vi "Check State.vi"(8 "error in (no error)":errorcluster, 11 "Shutter in":refnum<class "Shutter.lvclass">) -> (0 "error out":errorcluster, 3 "Shutter out":refnum<class "Shutter.lvclass">)   [LabVIEW 2016]
uses:
  Shutter.lvclass
  Controls/Shutter States.ctl
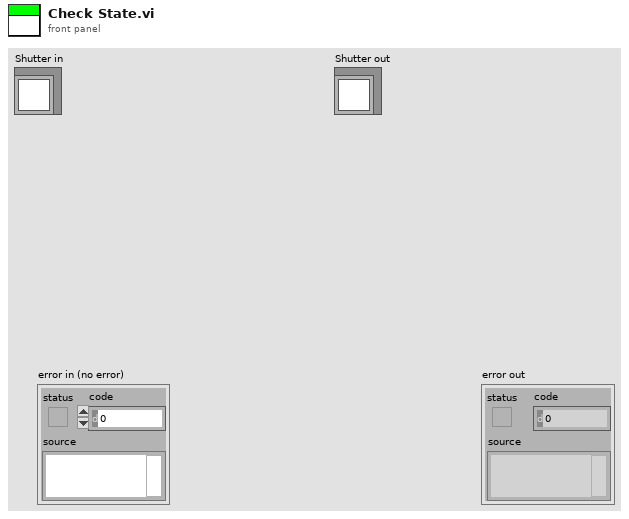
[diagram p1: front panel]
types:
  T1 = typedef "Shutter States.ctl" = enum16{"Open", "Close", "Wait", "Off", "Arm", "Idle"}
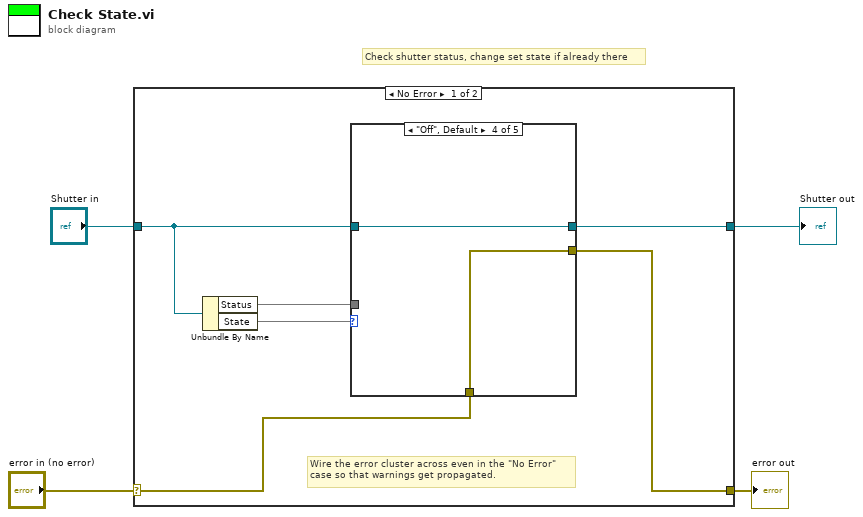
[diagram p0: block diagram]
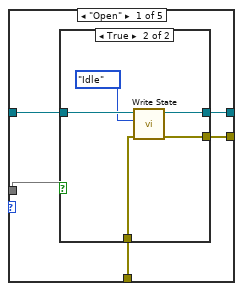
[diagram p2: hidden frame]
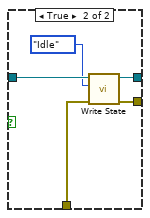
[diagram p5: hidden frame]
diagram:
  # "Check shutter status, change set state if already there"
  n1 = case shown="No Error" "error in (no error)" {
    selector: "error in (no error)" -> [w7 w38]
    tunnel: [w6 w38] -> w3
    tunnel: [w5 w37] -> w1
    tunnel: "Shutter in" -> [w8 w37]
    frame No Error {
      # "Wire the error cluster across even in the \"No Error\"\ncase so that warnings get propagated."
      n2 = Unbundle By Name(w8) -> ("Status"=w9, "State"=w10)
      n3 = case shown="\"Off\", Default" w10 {
        tunnel: w9 -> [w15 w27 _ _ _]
        tunnel: w8 -> [w14 w26 _ w36 _]
        tunnel: w7 -> [w13 w24 _ w35 _]
        tunnel: [w12 w23 _ w35 _] -> w6
        tunnel: [w11 w25 _ w36 _] -> w5
        frame "Open" {
          n4 = case shown="True" w15 {
            tunnel: w14 -> [w16 w22]
            tunnel: w13 -> [w17 w20]
            tunnel: [w17 w19] -> w12
            tunnel: [w16 w18] -> w11
            frame False {
            }
            frame True {
              n5 = call-dynamic "Write State.vi"("error in (no error)"=w20, "Set"=Shutter_States."Idle", "Shutter in"=w22) -> ("error out"=w19:errorcluster, "Shutter out"=w18:refnum<class "Shutter.lvclass">)  [unwired: 7 in]
            }
          }
        }
        frame "Close" {
          n6 = case shown="False" w27 {
            tunnel: w26 -> [w29 w34]
            tunnel: [w29 w33] -> w25
            tunnel: w24 -> [w28 w31]
            tunnel: [w28 w30] -> w23
            frame False {
            }
            frame True {
              n7 = call-dynamic "Write State.vi"("error in (no error)"=w31, "Set"=Shutter_States."Idle", "Shutter in"=w34) -> ("error out"=w30:errorcluster, "Shutter out"=w33:refnum<class "Shutter.lvclass">)  [unwired: 7 in]
            }
          }
        }
        frame "Wait" {
        }
        frame "Off", Default {
        }
        frame "Arm" {
        }
      }
    }
    frame Error {
    }
  }
  "error out" <- w3
  "Shutter out" <- w1
